vi "getItemType.vi"(8 "error in (no error)":errorcluster, 11 "IProperty in":refnum<class "IProperty.lvclass">) -> (0 "error out":errorcluster, 2 "Item Type out":T1 items=["ctBool"=0, "ctInt"=1, "ctFloat"=2, "ctString"=3, "ctList"=4, "ctDict"=5, "ctRatio"=6, "ctProc"=7, "ctObject"=8, "ctBinaryData"=9, "ctFunc"=10, "ctComplexNumber"=11, "ctStruct"=12, "ctEnumeration"=13, "ctUndefined"=65535], 3 "IProperty out":refnum<class "IProperty.lvclass">)   [LabVIEW 2022 SP3, in "openDAQ.lvlib" / "IBaseObject.lvlib" / "IProperty.lvlib" / "IProperty.lvclass"]
uses:
  <instrlib>/openDAQ/Public/Classes/IProperty/IProperty.lvclass
  C:/Program Files (x86)/National Instruments/LabVIEW 2022/instr.lib/openDAQ/Public/Classes/IBaseObject/IBaseObject.lvclass
  <instrlib>/openDAQ/Public/TypeDef/CoreType.ctl
  <instrlib>/openDAQ/Public/Classes/IBaseObject/IBaseObject.lvclass/IBaseObject.ctl
  <instrlib>/openDAQ/Public/Classes/IBaseObject/Accessor/Read reference.vi
  <instrlib>/openDAQ/Binaries/Windows/x86/copendaq32.dll
  <instrlib>/openDAQ/openDAQ.lvlib
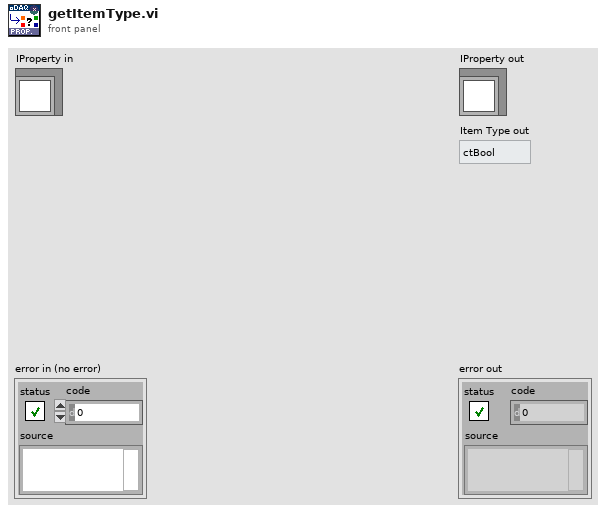
[diagram p1: front panel]
types:
  T1 = typedef "openDAQ.lvlib/CoreType.ctl" = u16
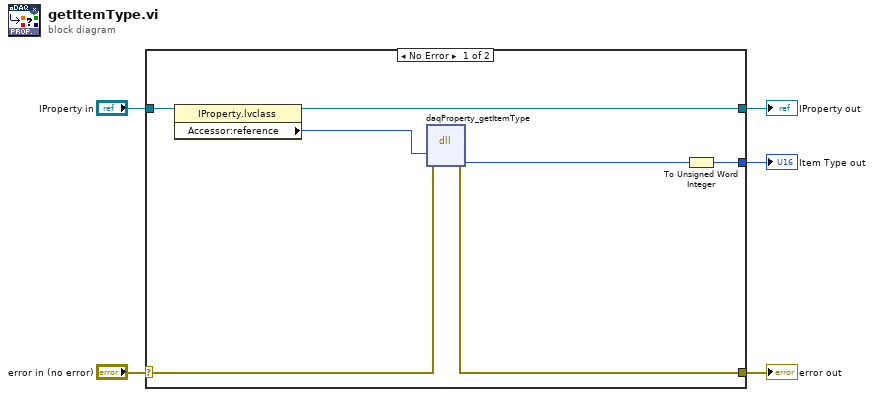
[diagram p0: block diagram]
diagram:
  n1 = case shown="No Error" "error in (no error)" {
    selector: "error in (no error)" -> [w11 w14]
    tunnel: [w10 w14] -> w4
    tunnel: [w9 w13] -> w2
    tunnel: "IProperty in" -> [w12 w13]
    tunnel: [w6 _] -> w1
    frame No Error {
      n2 = property class="IProperty.lvclass"(reference=w12) -> (reference out=w9:refnum<class "IProperty.lvclass">, "Accessor:reference"=w8:i64)  [unwired: 1 in, 1 out]
      n3 = dll-call lib="C:/Program Files (x86)/National Instruments/LabVIEW 2022/instr.lib/openDAQ/Binaries/Windows/x86/copendaq*.*" fn="daqProperty_getItemType"(error in=w11, "property"=w8) -> (error out=w10:errorcluster, "type"=w7:i64)  [unwired: 5 in, 1 out]
      n4 = To Unsigned Word Integer(number=w7) -> (unsigned 16bit integer=w6:u16)
    }
    frame Error {
    }
  }
  "error out" <- w4
  "IProperty out" <- w2
  "Item Type out" <- w1
